vi "Teleop.vi"(10 "Match Info":T1={"Autonomous Elapsed Seconds"=0.0, "TeleOp Elapsed Seconds"=0.0, "Disabled Elapsed Seconds"=0.0, "Visited Autonomous"=FALSE, "Visited TeleOp"=FALSE, "Visited Disabled"=FALSE, "Autonomous Settings"={"Autonomous Style"=enum."Independent", "VI Refnum"=refnum}}, 11 "Call Context":T2) -> ()   [LabVIEW 2015]
doc: "This VI is called for each TeleOp packet received from the DS where the robot is not disabled. It is often used to read from the joysticks and update I/O or to update setpoints for timed control loops. It should complete and return within 20 milliseconds or it may miss DS packets."
uses:
  <vilib>/Rock Robotics/WPI/DriverStation/WPI_DriverStationDerivedRobotMode.ctl
  <vilib>/Rock Robotics/WPI/DriverStation/WPI_DriverStationMatch Info.ctl
  <vilib>/Rock Robotics/WPI/Utilities/WPI_GetSetVariantRefNum.vi
  <vilib>/Rock Robotics/Network Tables/SD Write Boolean Array.vi
  <vilib>/Rock Robotics/Network Tables/SD Write Numeric Array.vi
  <vilib>/Rock Robotics/Network Tables/SD Read Number.vi
  <vilib>/Rock Robotics/Network Tables/SD Read Boolean.vi
  <vilib>/Rock Robotics/Network Tables/SD Write Number.vi
  <vilib>/Analysis/NI_AALPro.lvlib
panel:
  out "Distance":dbl
  out "Waveform Chart 2":dbl(graph)
  out "Waveform Chart":dbl(graph)
  out "Best Power Fit":dbl[](array[numeric])
  in  "fw speed":dbl(slide) scale=0.0..0.9
  out "Boolean":bool
  out "Sample Slider 0":dbl(slide) scale=0.0..5.0
  out "Sample Boolean 1":bool
  out "Sample Boolean 0":bool
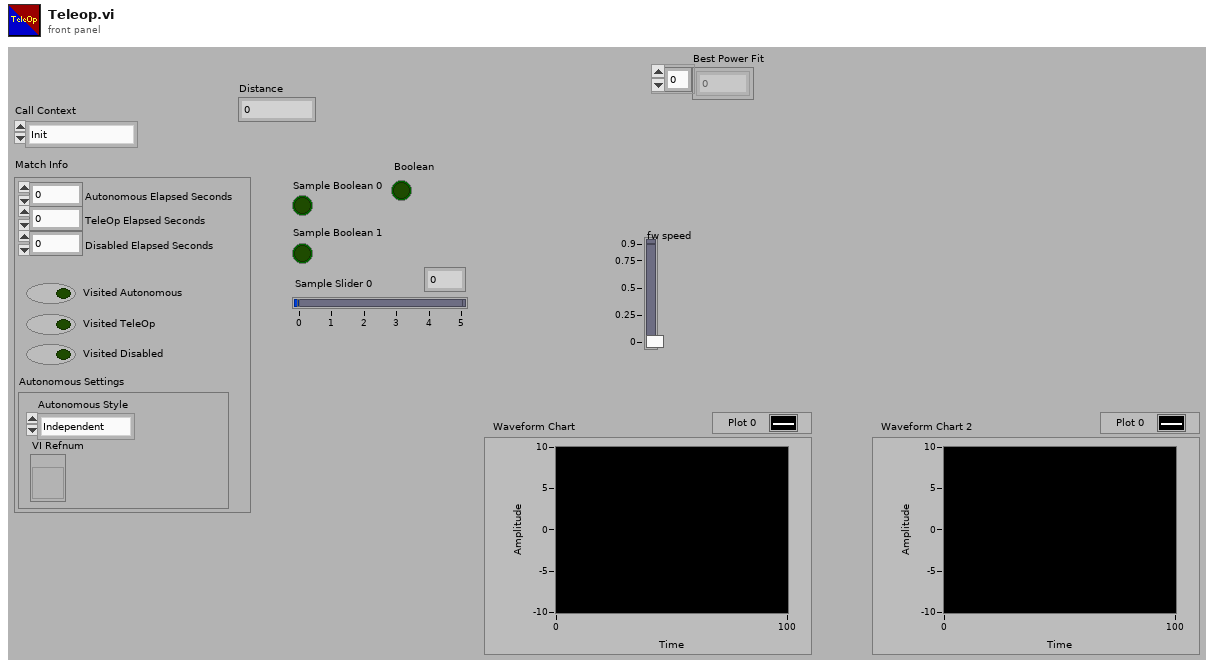
[diagram p1: front panel]
types:
  T1 = typedef "WPI_DriverStationMatch Info.ctl" = cluster{"Autonomous Elapsed Seconds":dbl, "TeleOp Elapsed Seconds":dbl, "Disabled Elapsed Seconds":dbl, "Visited Autonomous":bool, "Visited TeleOp":bool, "Visited Disabled":bool, "Autonomous Settings":cluster{"Autonomous Style":enum16{"Iterative", "Independent"}, "VI Refnum":refnum<vi>}}
  T2 = typedef "WPI_DriverStationDerivedRobotMode.ctl" = enum16{"Init", "Execute", "Stop"}
  T3 = typedef "WPI_JoystickDevRef.ctl" = cluster{"Device":T4}
  T4 = typedef "WPI_JoystickDeviceEnum.ctl" = enum16{"USB 0", "USB 1", "USB 2", "USB 3", "USB 4", "USB 5"}
  T5 = typedef "WPI_MotorControlDeviceRef.ctl" = cluster{"DeviceStatus":errorcluster, "Type":T6, "PWM":cluster{"PWM Channel":T7, "DeadBand":T8}, "CAN":cluster{"Device Number":u8, "Control Mode":T9, "Semaphore":T10, "Max Vout":dbl, "TalonSRX Control Mode":T11}, "Invert":bool}
  T6 = typedef "WPI_MotorControlType.ctl" = enum16{"PWM", "CAN", "CANTalonSRX"}
  T7 = typedef "FPGA_DIOPWMChannel.ctl" = enum8{"PWM 0", "PWM 1", "PWM 2", "PWM 3", "PWM 4", "PWM 5", "PWM 6", "PWM 7", "PWM 8", "PWM 9", "PWM MXP 0", "PWM MXP 1", "PWM MXP 2", "PWM MXP 3", "PWM MXP 4", "PWM MXP 5", "PWM MXP 6", "PWM MXP 7", "PWM MXP 8", "PWM MXP 9", "Invalid"}
  T8 = typedef "WPI_PWMDeadband.ctl" = cluster{"Name":string, "maxPositivePwm":i32, "minPositivePwm":i32, "centerPwm":i32, "maxNegativePwm":i32, "minNegativePwm":i32, "angularRange":u16}
  T9 = typedef "WPI_CANJaguar_ControlMode.ctl" = enum8{"Percent VBus", "Current", "Speed", "Position", "Voltage"}
  T10 = typedef "Semaphore RefNum" = refnum<k1>
  T11 = typedef "WPI_CANTalonSRX_APIControlMode.ctl" = enum8{"Percent VBus", "Speed", "Position", "Slave", "Unchanged / Invalid", "Voltage Compensation", "Current", "Motion Profile"}
  T12 = typedef "WPI_RobotDriveDevRef.ctl" = cluster{"DevStatus":errorcluster, "Motors[]":T5[], "Square Inputs":bool, "Max Output":dbl}
  T13 = typedef "WPI_EncoderDevRef.ctl" = cluster{"DevStatus":errorcluster, "EncoderIndex":T14, "CounterIndex":T15, "DistancePerCount":dbl, "Decoding Type":T16}
  T14 = typedef "FPGA_EncoderIdx.ctl" = enum8{"Enc 0", "Enc 1", "Enc 2", "Enc 3", "Enc 4", "Enc 5", "Enc 6", "Enc 7", "Invalid"}
  T15 = typedef "FPGA_CounterCtrSystemIndex.ctl" = enum8{"Ctr 0", "Ctr 1", "Ctr 2", "Ctr 3", "Ctr 4", "Ctr 5", "Ctr 6", "Ctr 7", "Invalid"}
  T16 = typedef "WPI_EncoderType.ctl" = enum16{"1x", "2x", "4x"}
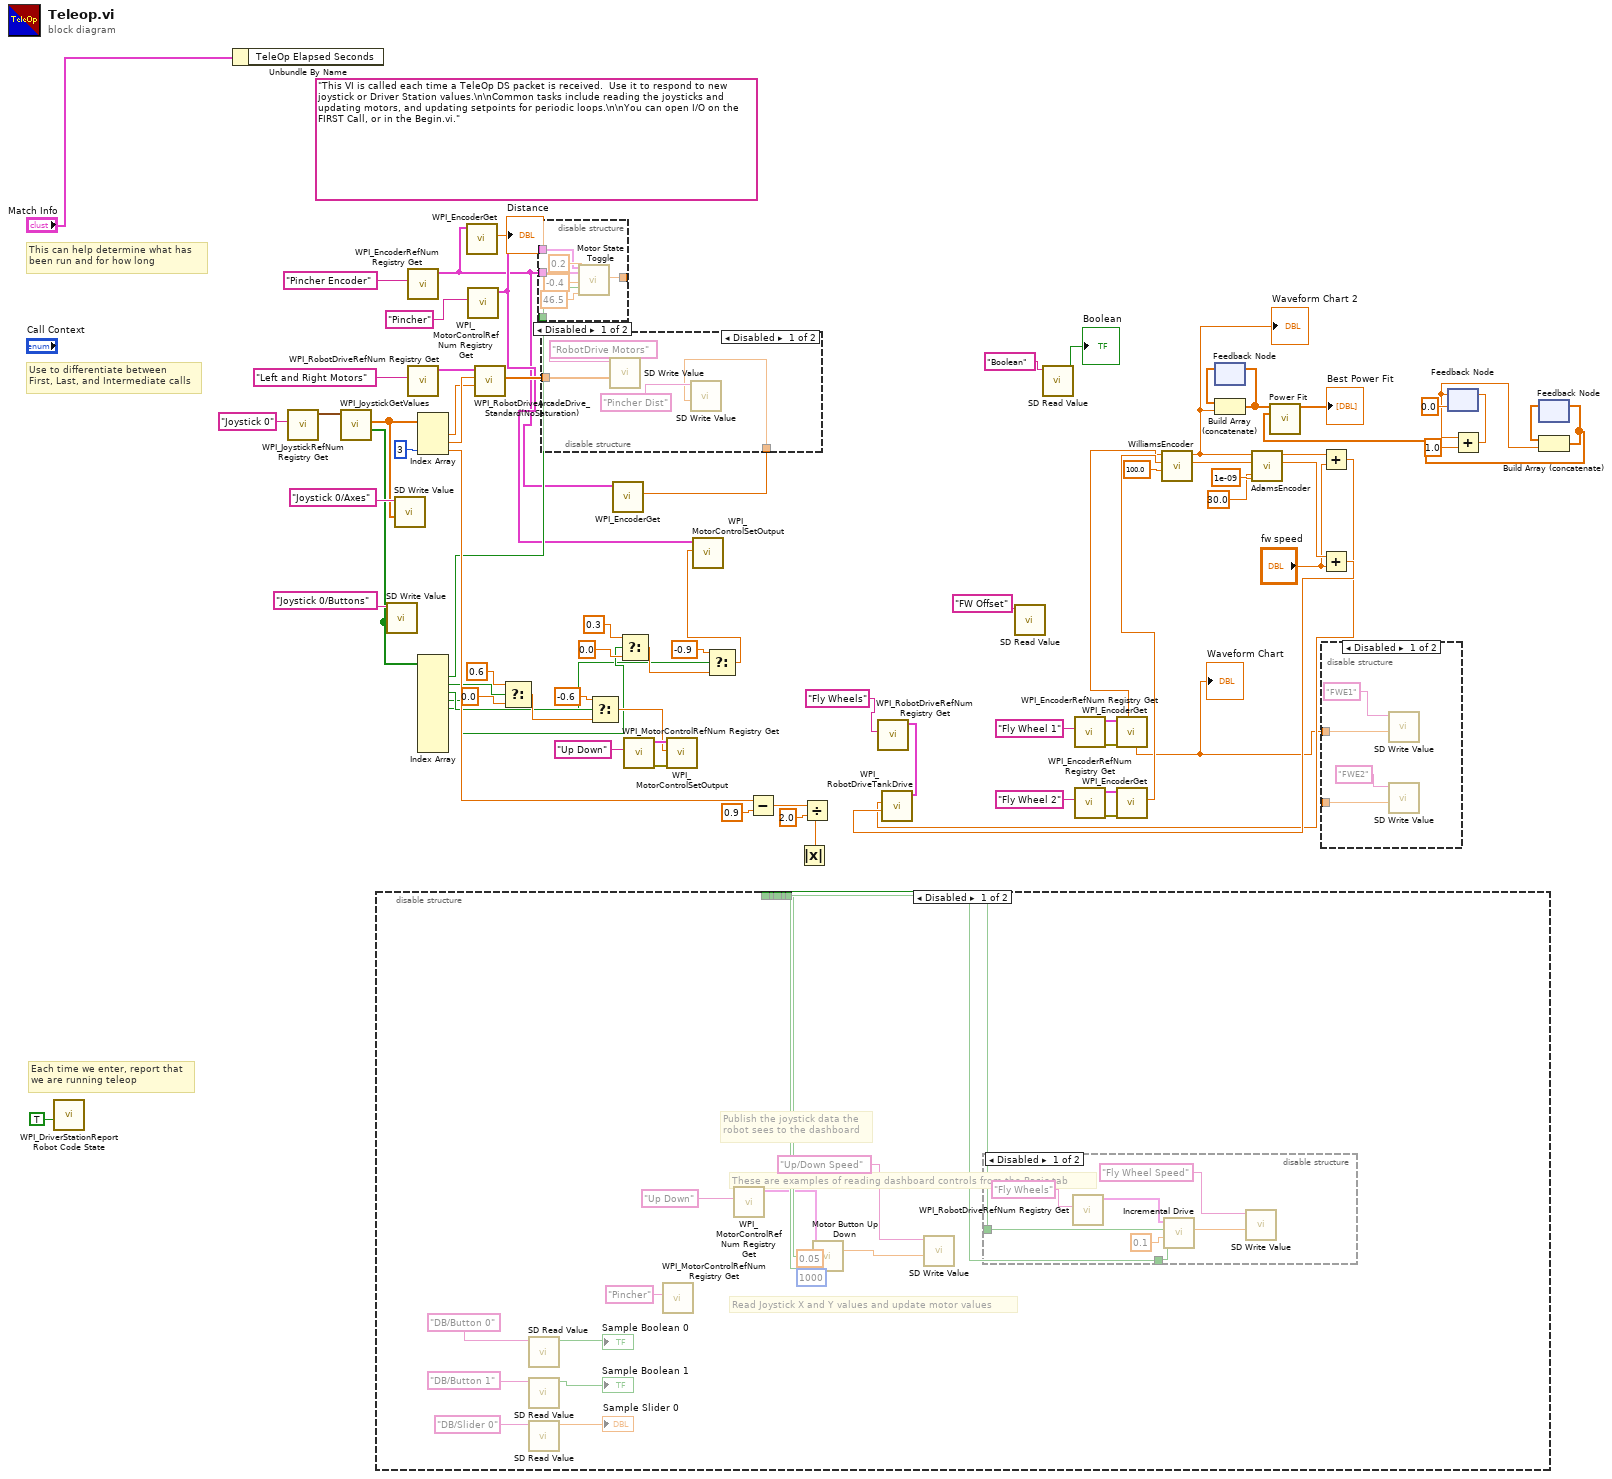
[diagram p0: block diagram]
diagram:
  (unwired) "This VI is called each time a TeleOp DS packet is received.  Use it to respond to new joystick or Driver Station values.\n\nCommon tasks include reading the joysticks and updating motors, and updating setpoints for periodic loops.\n\nYou can open I/O on the FIRST Call, or in the Begin.vi."
  # "Each time we enter, report that\nwe are running teleop"
  # "Use to differentiate between\nFirst, Last, and Intermediate calls"
  # "This can help determine what has\nbeen run and for how long"
  n1 = call <vilib>:"WPI_DriverStationReport Robot Code State.vi"("TeleOp"=TRUE ("Autonomous")) -> ()  [unwired: 10 in, 1 out]
  n2 = Unbundle By Name("Match Info") -> ()  [unwired: 1 out]
  n3 = call <vilib>:"WPI_JoystickRefNum Registry Get.vi"("refnum name"="Joystick 0") -> ("JoystickDevRef"=w72:T3)  [unwired: 1 in, 9 out]
  n4 = call <vilib>:"WPI_JoystickGetValues.vi"("JoystickDevRef"=w72) -> ("Buttons"=w65:bool[], "Axes"=w68:dbl[])  [unwired: 6 in, 3 out]
  n5 = disable-structure shown="Disabled" {
    disable-tunnel: _ -> [w88 _]
    disable-tunnel: _ -> [w87 _]
    disable-tunnel: _ -> [w83 _]
    disable-tunnel: _ -> [w82 _]
    disable-tunnel: _ -> [w78 _]
    frame Disabled {
      # "These are examples of reading dashboard controls from the Basic tab"
      # "Publish the joystick data the\nrobot sees to the dashboard"
      # "Read Joystick X and Y values and update motor values"
      n6 = call-poly <vilib>:"SD Read Value.vi"("Name"="DB/Button 0" ("refnum name")) -> ("Boolean"=→"Sample Boolean 0":bool)  [unwired: 8 in, 2 out]
      n7 = call-poly <vilib>:"SD Read Value.vi"("Name"="DB/Button 1" ("refnum name")) -> ("Boolean"=→"Sample Boolean 1":bool)  [unwired: 8 in, 2 out]
      n8 = call-poly <vilib>:"SD Read Value.vi"("Name"="DB/Slider 0" ("refnum name")) -> ("Numeric"=→"Sample Slider 0":dbl)  [unwired: 8 in, 2 out]
      n9 = call <vilib>:"WPI_MotorControlRefNum Registry Get.vi"("refnum name"="Pincher") -> ("MotorControlDevRef"=w79:T5)  [unwired: 9 in, 1 out]
      n10 = call <vilib>:"WPI_MotorControlRefNum Registry Get.vi"("refnum name"="Up Down") -> ("MotorControlDevRef"=w80:T5)  [unwired: 9 in, 1 out]
      n11 = call "Motor Button Up Down.vi"("MotorControlDevRef"=w80, "Min Time"=u64 1000, "Go Up"=w83, "Speed"=0.05 ("# Change Each Time"), "Go Down"=w82) -> ("Value Output"=w85:dbl)  [unwired: 10 in]
      n12 = call-poly <vilib>:"SD Write Value.vi"("Numeric"=w85, "Name"="Up/Down Speed") -> ()  [unwired: 8 in, 2 out]
      n13 = disable-structure shown="Disabled" {
        disable-tunnel: w88 -> [w99 _]
        disable-tunnel: w87 -> [w98 _]
        frame Disabled {
          n14 = call <vilib>:"WPI_RobotDriveRefNum Registry Get.vi"("refnum name"="Fly Wheels") -> ("RobotDriveDevRef"=w101:T12)  [unwired: 9 in, 1 out]
          n15 = call "Incremental Drive.vi"("Down Incremental"=w98, "# Change Each Time"=0.1, "Up Incremental"=w99, "RobotDriveDevRef"=w101) -> ("Value Out"=w97:dbl)  [unwired: 7 in]
          n16 = call-poly <vilib>:"SD Write Value.vi"("Numeric"=w97, "Name"="Fly Wheel Speed") -> ()  [unwired: 8 in, 2 out]
        }
        frame Enabled {
        }
      }
    }
    frame Enabled {
    }
  }
  n17 = call-poly <vilib>:"SD Write Value.vi"("Boolean Array"=w65, "Name"="Joystick 0/Buttons") -> ()  [unwired: 8 in, 2 out]
  n18 = call-poly <vilib>:"SD Write Value.vi"("Numeric Array"=w68, "Name"="Joystick 0/Axes") -> ()  [unwired: 8 in, 2 out]
  n19 = call <vilib>:"WPI_EncoderRefNum Registry Get.vi"("refnum name"="Pincher Encoder") -> ("EncoderDevRef"=w2:T13)  [unwired: 9 in, 1 out]
  n20 = call <vilib>:"WPI_RobotDriveRefNum Registry Get.vi"("refnum name"="Left and Right Motors") -> ("RobotDriveDevRef"=w74:T12)  [unwired: 1 in, 9 out]
  n21 = Index Array(array=w68, index #3=3 ("index")) -> (element #1=w63:dbl, element #2=w64:dbl, element #3=w62:dbl)  [unwired: 2 in]
  n22 = Index Array(array=w65) -> (element #1=w50:bool, element #2=w53:bool, element #3=w52:bool, element #4=w37:bool, element #5=w36:bool)  [unwired: 10 in, 5 out]
  n23 = call <vilib>:"WPI_EncoderGet.vi"("EncoderDevRef"=w2) -> ("Distance"=→"Distance":dbl)  [unwired: 5 in, 5 out]
  n24 = call <vilib>:"WPI_MotorControlRefNum Registry Get.vi"("refnum name"="Pincher") -> ("MotorControlDevRef"=w33:T5)  [unwired: 9 in, 1 out]
  n25 = call <vilib>:"WPI_RobotDriveArcadeDrive_Standard(NoSaturation).vi"("Y axis value"=w63, "X axis value"=w64, "RobotDriveDevRef"=w74) -> ("Motor Values"=w70:dbl[])  [unwired: 1 in, 7 out]
  n26 = Select(t=0.6, s=w53, f=0.0) -> (s? t:f=w58:dbl)
  n27 = disable-structure shown="Disabled" {
    disable-tunnel: w50 -> [w109 _]
    disable-tunnel: w2 -> [w108 _]
    disable-tunnel: [w104 _] -> _
    disable-tunnel: w33 -> [w103 _]
    frame Disabled {
      n28 = call "Motor State Toggle.vi"("MotorControlDevRef"=w103, "EncoderDevRef"=w108, "Upper Limit"=0.2, "Motor Speed"=-0.4, "Switch States"=w109, "Lower Limit"=46.5) -> ("Distance"=w104:dbl)  [unwired: 11 in, 2 out]
    }
    frame Enabled {
    }
  }
  n29 = Select(t=-0.6, s=w52, f=w58) -> (s? t:f=w55:dbl)
  n30 = call <vilib>:"WPI_EncoderGet.vi"("EncoderDevRef"=w2) -> ("Distance"=w35:dbl)  [unwired: 5 in, 5 out]
  n31 = disable-structure shown="Disabled" {
    disable-tunnel: w70 -> [w112 _]
    disable-tunnel: w35 -> [w110 _]
    frame Disabled {
      n32 = call-poly <vilib>:"SD Write Value.vi"("Numeric Array"=w112, "Name"="RobotDrive Motors") -> ()  [unwired: 8 in, 2 out]
      n33 = call-poly <vilib>:"SD Write Value.vi"("Numeric"=w110, "Name"="Pincher Dist") -> ()  [unwired: 8 in, 2 out]
    }
    frame Enabled {
    }
  }
  n34 = Select(t=0.3, s=w37, f=0.0) -> (s? t:f=w40:dbl)
  n35 = call <vilib>:"WPI_MotorControlRefNum Registry Get.vi"("refnum name"="Up Down") -> ("error out"=w61:errorcluster, "MotorControlDevRef"=w60:T5)  [unwired: 9 in]
  n36 = call <vilib>:"WPI_MotorControlSetOutput.vi"("error in (no error)"=w61, "Output"=w55, "MotorControlDevRef"=w60) -> ()  [unwired: 6 in, 3 out]
  n37 = Select(t=-0.9, s=w36, f=w40) -> (s? t:f=w34:dbl)
  n38 = call <vilib>:"WPI_MotorControlSetOutput.vi"("Output"=w34, "MotorControlDevRef"=w33) -> ()  [unwired: 7 in, 3 out]
  n39 = Subtract(x=w62, y=0.9) -> (x-y=w45:dbl)
  n40 = Divide(x=w45, y=2.0) -> (x/y=w44:dbl)
  n41 = Absolute Value(x=w44) -> ()  [unwired: 1 out]
  n42 = call <vilib>:"WPI_RobotDriveRefNum Registry Get.vi"("refnum name"="Fly Wheels") -> ("RobotDriveDevRef"=w48:T12)  [unwired: 9 in, 1 out]
  n43 = call-poly <vilib>:"SD Read Value.vi"("Name"="FW Offset") -> ()  [unwired: 8 in, 3 out]
  n44 = call-poly <vilib>:"SD Read Value.vi"("Name"="Boolean") -> ("Boolean"=→"Boolean":bool)  [unwired: 8 in, 2 out]
  n45 = call <vilib>:"WPI_EncoderRefNum Registry Get.vi"("refnum name"="Fly Wheel 1") -> ("error out"=w32:errorcluster, "EncoderDevRef"=w25:T13)  [unwired: 9 in]
  n46 = call <vilib>:"WPI_EncoderRefNum Registry Get.vi"("refnum name"="Fly Wheel 2") -> ("error out"=w30:errorcluster, "EncoderDevRef"=w29:T13)  [unwired: 9 in]
  n47 = call <vilib>:"WPI_EncoderGet.vi"("error in (no error)"=w32, "EncoderDevRef"=w25) -> ("Distance"=w6:dbl, "Rate"=w5:dbl)  [unwired: 4 in, 4 out]
  "Waveform Chart" <- w5
  n48 = call <vilib>:"WPI_EncoderGet.vi"("error in (no error)"=w30, "EncoderDevRef"=w29) -> ("Distance"=w7:dbl)  [unwired: 4 in, 5 out]
  n49 = call "WilliamsEncoder.vi"("Delta T"=100.0, "Distance 2"=w7, "Distance 1"=w6) -> ("Rate 2"=w3:dbl, "Rate 1"=w4:dbl)  [unwired: 7 in]
  "Waveform Chart 2" <- w4
  n50 = feedback #1() -> (w14:dbl[])  [unwired: 1 in]
  n51 = Build Array (concatenate)(w14, w4) -> (w15:dbl[])
  n52 = feedback-in #1(w15) -> ()
  n53 = call "AdamsEncoder.vi"("DiffConstant"=30.0, "Change each time"=1e-09, "FW2Rate"=w3, "FW1Rate"=w4) -> ("FW2Change"=w18:dbl, "FW1Change"=w19:dbl)  [unwired: 6 in]
  n54 = Add(x=w19, y="fw speed") -> (x+y=w20:dbl)
  n55 = Add(x=w18, y="fw speed") -> (x+y=w21:dbl)
  n56 = call <vilib>:"WPI_RobotDriveTankDrive.vi"("Right axis value"=w21, "Left axis value"=w20, "RobotDriveDevRef"=w48) -> ()  [unwired: 6 in, 3 out]
  n57 = disable-structure shown="Disabled" {
    disable-tunnel: w5 -> [w115 _]
    disable-tunnel: _ -> [w114 _]
    frame Disabled {
      n58 = call-poly <vilib>:"SD Write Value.vi"("Numeric"=w115, "Name"="FWE1") -> ()  [unwired: 8 in, 2 out]
      n59 = call-poly <vilib>:"SD Write Value.vi"("Numeric"=w114, "Name"="FWE2") -> ()  [unwired: 8 in, 2 out]
    }
    frame Enabled {
    }
  }
  n60 = feedback #2(0.0) -> (w9:dbl)
  n61 = Add(x=w9, y=1.0) -> (x+y=w13:dbl)
  n62 = feedback-in #2(w13) -> ()
  n63 = feedback #3() -> (w10:dbl[])  [unwired: 1 in]
  n64 = Build Array (concatenate)(w10, w9) -> (w8:dbl[])
  n65 = call <vilib>:"Power Fit.vi"("Y"=w15, "X"=w8) -> ("Best Power Fit"=→"Best Power Fit":dbl[])  [unwired: 8 in, 5 out]
  n66 = feedback-in #3(w8) -> ()
